vi "WSVCAP SHL Host LL Manage FPGA Top Level Controls Manage Instance IDs.vi"(0 "FPGA":T3, 11 "error in (no error)":errorcluster, 12 "Operation":T2) -> (4 "VI Ref":T1, 15 "error out":errorcluster)   [LabVIEW 2012]
uses:
  Type Defs/WSVCAP SHL I2C FPGA Enum.ctl
  user.lib/Utilities/Type Defs/MISC Instance Manager Operation.ctl
  Type Defs/WSVCAP SHL Manage FPGA Top Level Controls VI Ref.ctl
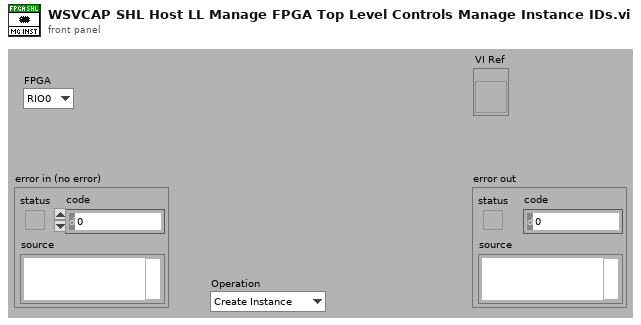
[diagram p1: front panel]
types:
  T1 = typedef "WSVCAP SHL Manage FPGA Top Level Controls VI Ref.ctl" = refnum<vi>
  T2 = typedef "MISC Instance Manager Operation.ctl" = enum16{"Create Instance", "Get Instance ID"}
  T3 = typedef "WSVCAP SHL I2C FPGA Enum.ctl" = enum16{"RIO0", "RIO1"}
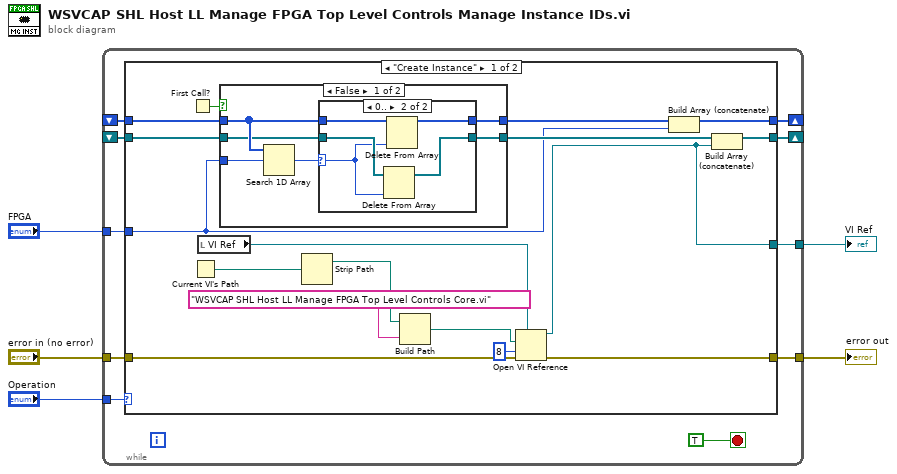
[diagram p0: block diagram]
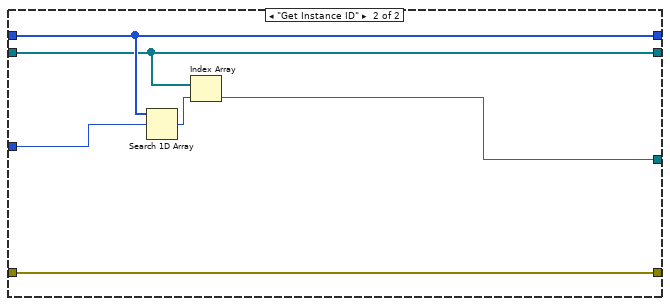
[diagram p4: hidden frame]
diagram:
  n1 = while {
    tunnel: "error in (no error)" -> [w15]
    tunnel: [w14] -> w4
    shift-right: [w8] -> _
    shift-left: _ -> [w11]
    shift-right: [w7] -> _
    shift-left: _ -> [w10]
    tunnel: "Operation" -> [w13]
    tunnel: "FPGA" -> [w9]
    tunnel: [w6] -> w1
    stop <- TRUE stop-if-true
    n2 = case shown="\"Create Instance\"" w13 {
      tunnel: w15 -> [w32 w47]
      tunnel: [w18 w47] -> w14
      tunnel: w11 -> [w29 w49]
      tunnel: w10 -> [w28 w48]
      tunnel: w9 -> [w25 w51]
      tunnel: [w31 w49] -> w8
      tunnel: [w21 w48] -> w7
      tunnel: [w17 w46] -> w6
      frame "Create Instance" {
        n3 = First Call?() -> (First Call?: T/F=w30:bool)
        n4 = Current VI's Path() -> (path=w22:path)
        n5 = local read "VI Ref"() -> (w16:T1)
        n6 = case shown="False" w30 {
          tunnel: w29 -> [w37 _]
          tunnel: w28 -> [w36 _]
          tunnel: [w34 _] -> w27
          tunnel: [w33 _] -> w26
          tunnel: w25 -> [w38 _]
          frame False {
            n7 = Search 1D Array(1D array=w37, element=w38) -> (index of element=w35:i32)  [unwired: 1 out]
            n8 = case shown="0.." w35 {
              selector: w35 -> [_ w41]
              tunnel: w37 -> [w40 w45]
              tunnel: w36 -> [w39 w44]
              tunnel: [w40 w43] -> w34
              tunnel: [w39 w42] -> w33
              frame Default {
              }
              frame 0.. {
                n9 = Delete From Array(array=w44, index=w41) -> (array with subset deleted=w42:T1[])  [unwired: 1 in, 1 out]
                n10 = Delete From Array(array=w45, index=w41) -> (array with subset deleted=w43:T3[])  [unwired: 1 in, 1 out]
              }
            }
          }
          frame True {
          }
        }
        n11 = Strip Path(path=w22) -> (stripped path=w19:path)  [unwired: 1 out]
        n12 = Build Path(base path=w19, name or relative path="WSVCAP SHL Host LL Manage FPGA Top Level Controls Core.vi" ("vi path")) -> (appended path=w20:path)
        n13 = Open VI Reference(type specifier VI Refnum (for type only)=w16, vi path=w20, options=8, error in (no error)=w32) -> (vi reference=w17:T1, error out=w18:errorcluster)  [unwired: 2 out]
        n14 = Build Array (concatenate)(w27, w25) -> (w31:T3[])
        n15 = Build Array (concatenate)(w26, w17) -> (w21:T1[])
      }
      frame "Get Instance ID" {
        n16 = Search 1D Array(1D array=w49, element=w51) -> (index of element=w50:i32)  [unwired: 1 out]
        n17 = Index Array(array=w48, index=w50) -> (element=w46:T1)
      }
    }
  }
  "error out" <- w4
  "VI Ref" <- w1
